vi "Send Message.vi"(8 "error in (no error)":errorcluster, 9 "Priority (Normal)":T1=enum."Normal", 10 "Message":refnum<class "Message.lvclass">, 11 "Actor API in":refnum<class "Actor API.lvclass">) -> (0 "error out":errorcluster, 3 "Actor API out":refnum<class "Actor API.lvclass">)   [LabVIEW 2020, in "Artifex.lvlib" / "Actor API.lvclass"]
uses:
  Actor API.lvclass
  Message/Message.lvclass
  Priority.ctl
  Actor API.lvclass/Actor API.ctl
  Priority Message Queue/Priority Message Queue.lvclass
  Artifex.lvlib
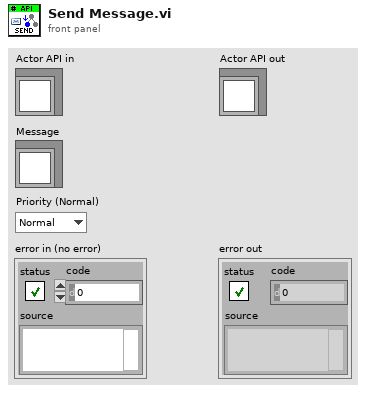
[diagram p1: front panel]
types:
  T1 = typedef "Artifex.lvlib/Priority.ctl" = enum16{"Low", "Normal", "High"}
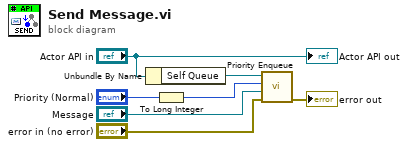
[diagram p0: block diagram]
diagram:
  n1 = Unbundle By Name("Actor API in") -> ("Self Queue"=w6:refnum<class "Priority Message Queue.lvclass">)
  n2 = To Long Integer(number="Priority (Normal)") -> (32bit integer=w4:i32)
  n3 = call "Priority Enqueue.vi"("error in (no error)"="error in (no error)", "Message"="Message", "Priority"=w4, "Priority Message Queue in"=w6) -> ("error out"=→"error out":errorcluster)  [unwired: 6 in, 1 out]
  "Actor API out" <- "Actor API in"
